vi "GetTreeChildren.vi"(8 "error in (no error)":errorcluster, 10 "name":string, 11 "Tree 2":refnum<vi>) -> (3 "Children":string[](array[string]))   [LabVIEW 2025]
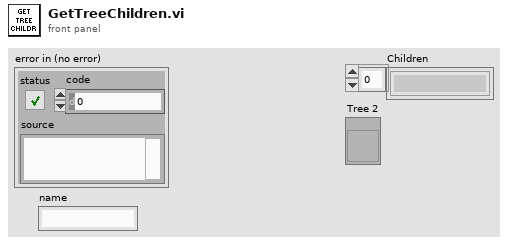
[diagram p1: front panel]
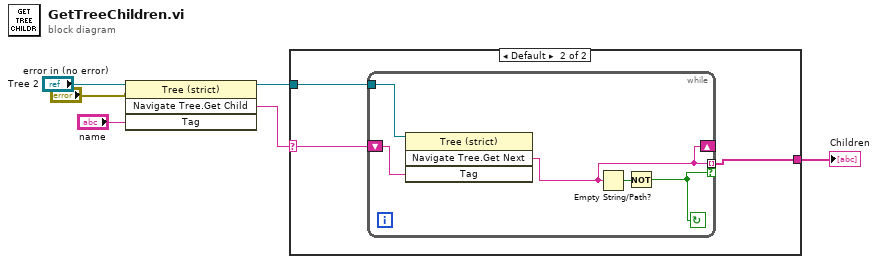
[diagram p0: block diagram]
diagram:
  n1 = invoke on="Invoke Node" class="Tree (strict)" method="Navigate Tree.Get Child"(reference="Tree 2", error in="error in (no error)", "Tag"="name") -> (reference out=w4:refnum<vi>, "Navigate Tree:Get Child"=w5:string)  [unwired: 1 in, 2 out]
  n2 = case shown="Default" w5 {
    selector: w5 -> [_ w9]
    tunnel: w4 -> [_ w8]
    tunnel: [_ w7] -> w3
    frame "" {
    }
    frame Default {
      n3 = while {
        shift-right: [w12] -> _
        shift-left: w9 -> [w13]
        tunnel: w8 -> [w14]
        tunnel: [w12] -> w7 mode=indexing if=w10
        stop <- w10 continue-if-true
        n4 = invoke class="Tree (strict)" method="Navigate Tree.Get Next"(reference=w14, "Tag"=w13) -> ("Navigate Tree:Get Next Item"=w12:string)  [unwired: 2 in, 3 out]
        n5 = Empty String/Path?(string/path=w12) -> (empty?=w11:bool)
        n6 = Not(x=w11) -> (.not. x?=w10:bool)
      }
    }
  }
  "Children" <- w3
